vi "AFM_Driver_Manager.GetPublicEvents.vi"(8 "error in (no error)":errorcluster, 11 "AFM_Driver_Manager in":refnum<class "AFM_Driver_Manager.lvclass">) -> (0 "error out":errorcluster, 2 "AFM_Driver Events":T1, 3 "AFM_Driver_Manager out":refnum<class "AFM_Driver_Manager.lvclass">)   [LabVIEW 2019, in "AFM_Driver_Manager.lvclass"]
uses:
  AFM_Driver_Manager.lvclass
  AFM_Driver_Manager.PublicEvents.ctl
  <userlib>/LevyLab/Relay Box/Typedefs/Resistor--enum.ctl
  AFM_Driver_Manager.lvclass/AFM_Driver_Manager.ctl
  <userlib>/LevyLab/Relay Box/Relay-Box.lvclass
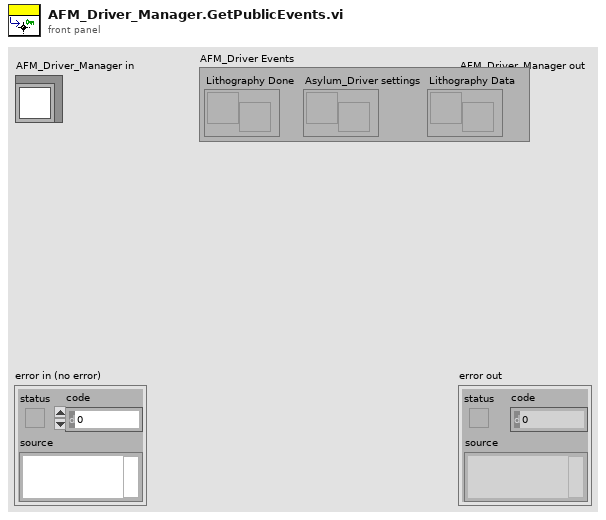
[diagram p1: front panel]
types:
  T1 = typedef "AFM_Driver_Manager.lvclass/AFM_Driver_Manager.PublicEvents.ctl" = cluster{"Lithography Done":refnum<user-event>, "Asylum_Driver settings":refnum<user-event>, "Lithography Data ":refnum<user-event>}
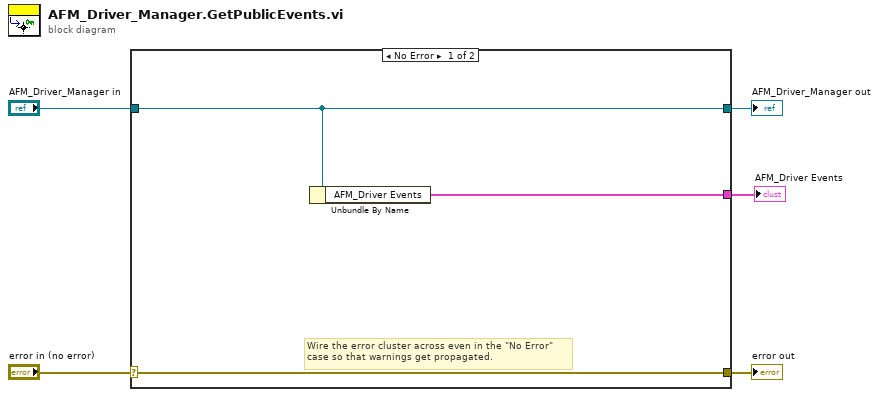
[diagram p0: block diagram]
diagram:
  n1 = case shown="No Error" "error in (no error)" {
    selector: "error in (no error)" -> [w8 w10]
    tunnel: [w8 w10] -> w4
    tunnel: [w7 w9] -> w2
    tunnel: "AFM_Driver_Manager in" -> [w7 w9]
    tunnel: [w6 _] -> w1
    frame No Error {
      # "Wire the error cluster across even in the \"No Error\"\ncase so that warnings get propagated."
      n2 = Unbundle By Name(w7) -> ("AFM_Driver Events"=w6:T1)
    }
    frame Error {
    }
  }
  "error out" <- w4
  "AFM_Driver_Manager out" <- w2
  "AFM_Driver Events" <- w1
